vi "Zedver_v3.vi"() -> ()   [LabVIEW 2011]
uses:
  Control 2.ctl
panel:
  out "Error":bool
  out "Datos recibidos (HEX)":string
  out "Bytes Procesado":u16
  out "Bytes Histograma":u16
  out "RAW Bytes":u16
  out "Com Cluster":T1
  out "Datos enviados (HEX)":string
  in  "Modo funcionamiento":T2="1"
  in  "PROCE CSV":path=path "D:/UV/IFIMED/LabVIEW/Excel_read/Excel2.csv"
  in  "HISTO CSV":path=path "D:/UV/IFIMED/LabVIEW/Excel_read/Excel2.csv"
  in  "RAW CSV":path=path "D:/UV/IFIMED/LabVIEW/Excel_read/Excel2.csv"
  in  "Histograma":bool
  in  "RAW":bool
  in  "Procesado":bool
  in  "Finalizar conexión":bool
  in  "Ejecutar petición":bool
  # "Ficheros simulación"
  # "Trabajo Fin de Grado\nGrado en Ingeniería Electrónica de Telecomunicación\nSistema de adquisición basado en FPGAs para \nlaboratorio de radiofrecuencia del Instituto de Física Médica."
  # "Autor:\n   Eladio Barrio Querol\nTutor externo: \n   Daniel Esperante Pereira\nTutor academico:\n   Vicente González Millán"
  # "Visualización respuesta y petición"
  # "Control comunicación"
  # "Datos de petición"
  # "Longitud en bytes"
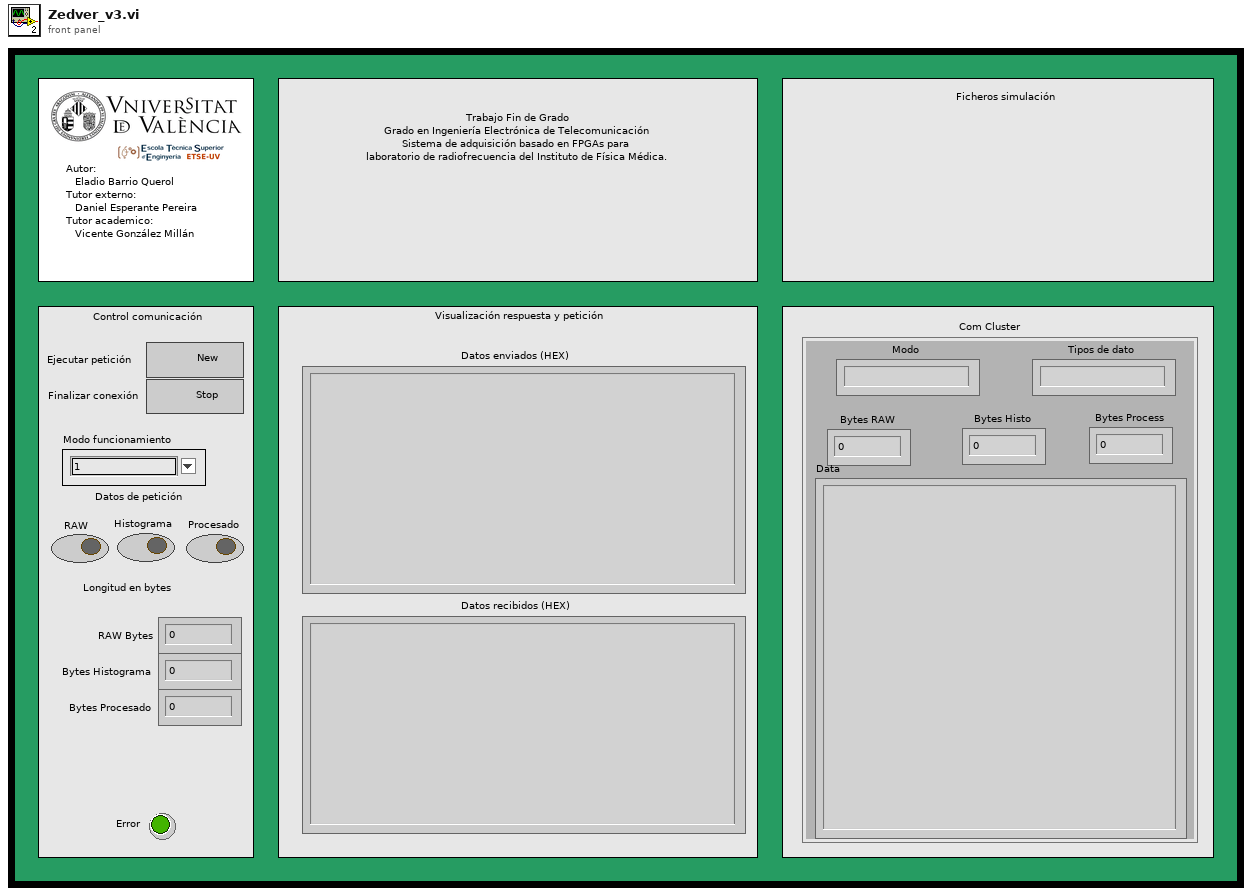
[diagram p1: front panel]
types:
  T1 = cluster{"Modo":string, "Tipos de dato":string, "Bytes RAW":u16, "Bytes Histo":u16, "Bytes Process":u16, "Data":string}
  T2 = typedef "Control 2.ctl" = string
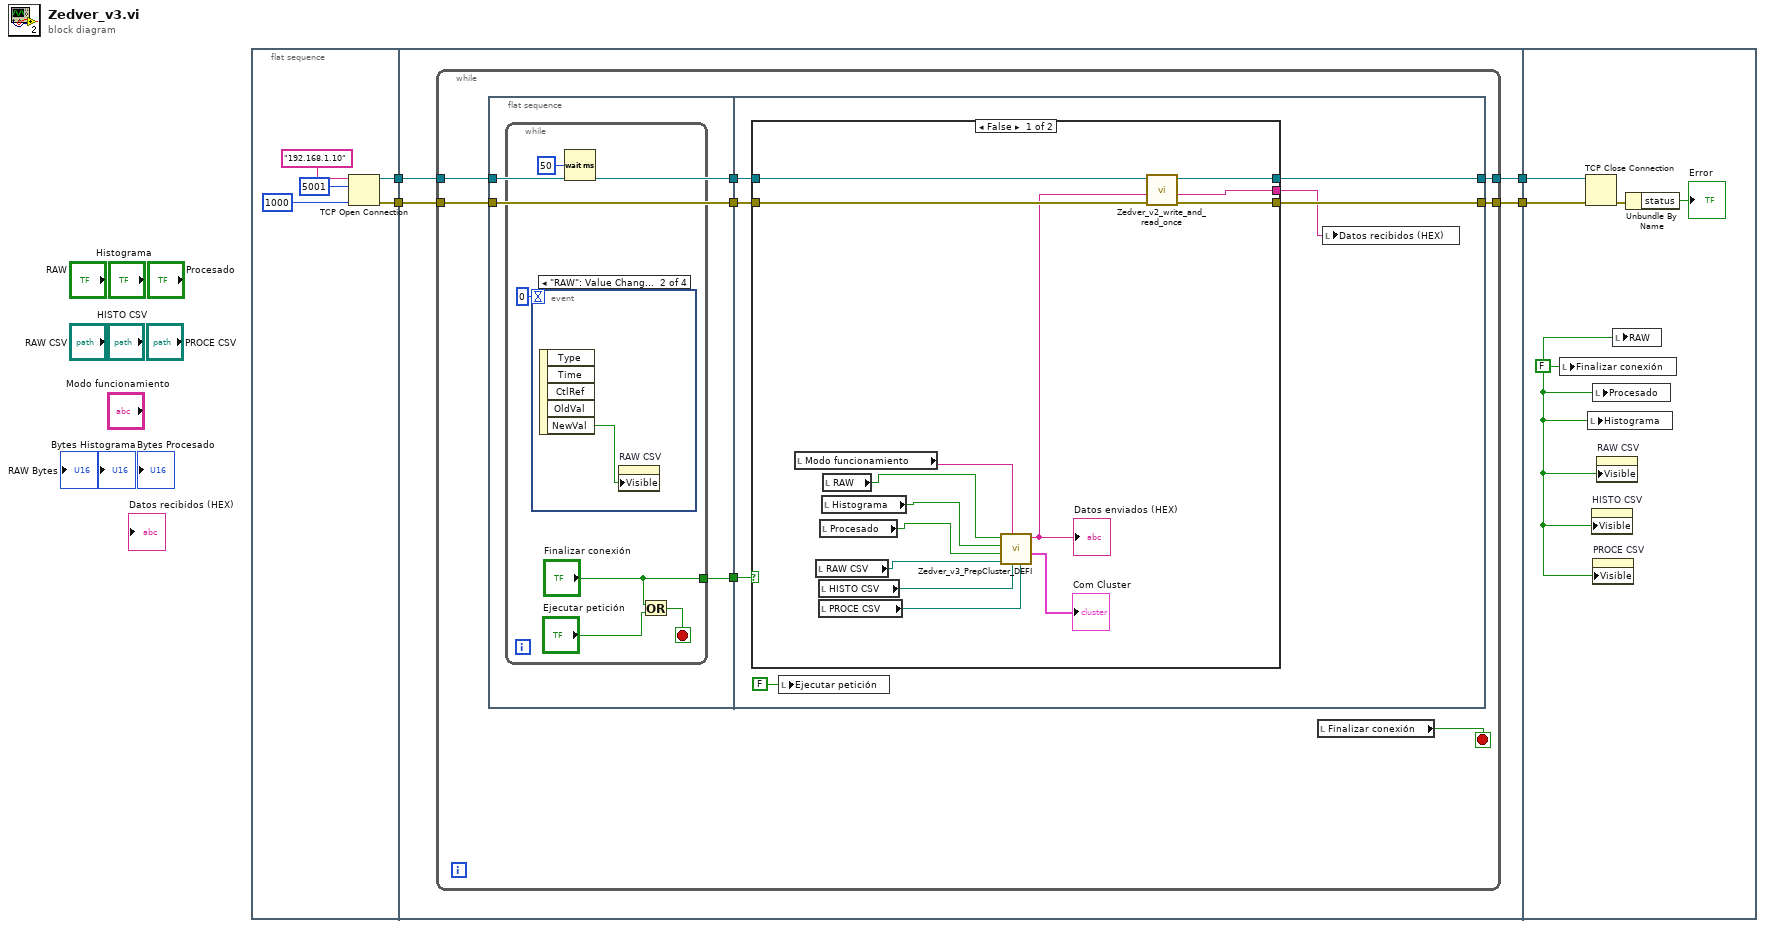
[diagram p0: block diagram]
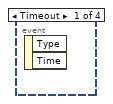
[diagram p2: hidden frame]
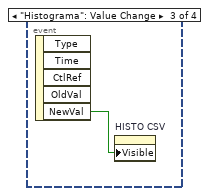
[diagram p3: hidden frame]
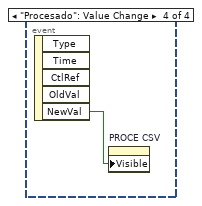
[diagram p4: hidden frame]
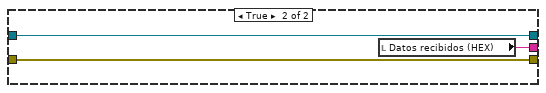
[diagram p5: hidden frame]
diagram:
  n1 = flat-sequence {
    tunnel: [w7] -> w4
    tunnel: [w6] -> w2
    tunnel: w4 -> [w13]
    tunnel: [w12] -> w3
    tunnel: w2 -> [w11]
    tunnel: [w10] -> w1
    tunnel: w3 -> [w60]
    tunnel: w1 -> [w59]
    frame #0 {
      n2 = TCP Open Connection(address="192.168.1.10", remote port or service name=u16 5001, timeout ms (60000)=1000) -> (connection ID=w7:refnum<k5>, error out=w6:errorcluster)  [unwired: 2 in]
    }
    frame #1 {
      n3 = while {
        tunnel: w13 -> [w19]
        tunnel: [w17] -> w12
        tunnel: w11 -> [w16]
        tunnel: [w14] -> w10
        stop <- w20 stop-if-true
        n4 = flat-sequence {
          tunnel: [w24] -> w21
          tunnel: w19 -> [w23]
          tunnel: [w23] -> w18
          tunnel: w16 -> [w22]
          tunnel: [w22] -> w15
          tunnel: w21 -> [w38]
          tunnel: w18 -> [w37]
          tunnel: [w36] -> w17
          tunnel: w15 -> [w33]
          tunnel: [w35] -> w14
          frame #0 {
            n5 = while {
              tunnel: ["Finalizar conexión"] -> w24
              stop <- w28 stop-if-true
              n6 = event shown="[1] \"RAW\": Value Change" {
                selector: _ -> [_ _ _ _]
                dyn-events: _ -> [_ _ _ _]
                timeout: 0 -> [_ _ _ _]
                event Timeout {
                  n7 = event-data() -> ()  [unwired: 1 in, 2 out]
                }
                event "RAW": Value Change {
                  n8 = event-data() -> ("NewVal"=w30:bool)  [unwired: 1 in, 4 out]
                  n9 = property on="RAW CSV" class="Path"("Visible"=w30) -> ()  [unwired: 2 in, 2 out]
                }
                event "Histograma": Value Change {
                  n10 = event-data() -> ("NewVal"=w31:bool)  [unwired: 1 in, 4 out]
                  n11 = property on="HISTO CSV" class="Path"("Visible"=w31) -> ()  [unwired: 2 in, 2 out]
                }
                event "Procesado": Value Change {
                  n12 = event-data() -> ("NewVal"=w32:bool)  [unwired: 1 in, 4 out]
                  n13 = property on="PROCE CSV" class="Path"("Visible"=w32) -> ()  [unwired: 2 in, 2 out]
                }
              }
              n14 = Wait (ms)(milliseconds to wait=u32 50) -> ()  [unwired: 1 out]
              n15 = Or(x="Finalizar conexión", y="Ejecutar petición") -> (x .or. y?=w28:bool)
            }
          }
          frame #1 {
            n16 = case shown="False" w38 {
              tunnel: w37 -> [w45 w56]
              tunnel: [w42 w56] -> w36
              tunnel: [w43 w55] -> w35
              tunnel: [w41 w54] -> w34
              tunnel: w33 -> [w44 w55]
              frame False {
                n17 = local read "Modo funcionamiento"() -> (w47:T2)
                n18 = local read "RAW CSV"() -> (w49:path)
                n19 = local read "HISTO CSV"() -> (w48:path)
                n20 = local read "PROCE CSV"() -> (w53:path)
                n21 = local read "Procesado"() -> (w50:bool)
                n22 = local read "Histograma"() -> (w51:bool)
                n23 = local read "RAW"() -> (w52:bool)
                n24 = call "Zedver_v3_PrepCluster_DEFI.vi"("PROCE CSV"=w53, "HISTO CSV"=w48, "Petición"=w47, "RAW CSV"=w49, "Procesado"=w50, "Histograma"=w51, "RAW"=w52) -> ("input cluster"=→"Com Cluster":T1, "data string"=w40:string)  [unwired: 3 in]
                "Datos enviados (HEX)" <- w40
                n25 = call "Zedver_v2_write_and_read_once.vi"("connection ID in"=w45, "data to send"=w40, "error in"=w44) -> ("connection ID out"=w42:refnum<k5>, "data read"=w41:string, "error out"=w43:errorcluster)  [unwired: 5 in]
              }
              frame True {
                n26 = local read "Datos recibidos (HEX)"() -> (w54:string)
              }
            }
            n27 = local write "Ejecutar petición"(FALSE ("New Button")) -> ()
            n28 = local write "Datos recibidos (HEX)"(w34) -> ()
          }
        }
        n29 = local read "Finalizar conexión"() -> (w20:bool)
      }
    }
    frame #2 {
      w61 = FALSE ("Finalizar conexión")
      n30 = local write "Finalizar conexión"(w61) -> ()
      n31 = TCP Close Connection(connection ID=w60, error in (no error)=w59) -> (error out=w58:errorcluster)  [unwired: 1 in, 1 out]
      n32 = local write "Histograma"(w61) -> ()
      n33 = property on="HISTO CSV" class="Path"("Visible"=w61) -> ()  [unwired: 2 in, 2 out]
      n34 = local write "Procesado"(w61) -> ()
      n35 = property on="PROCE CSV" class="Path"("Visible"=w61) -> ()  [unwired: 2 in, 2 out]
      n36 = property on="RAW CSV" class="Path"("Visible"=w61) -> ()  [unwired: 2 in, 2 out]
      n37 = local write "RAW"(w61) -> ()
      n38 = Unbundle By Name(w58) -> ("status"=→"Error":bool)
    }
  }
